vi "send_generic_trigger.vi"(7 "ensure unique insertion?":bool, 8 "error in (no error)":errorcluster, 9 "trigger type":T1, 10 "trigger variant":variant, 11 "GenericToplevelComponent in":refnum<class "GenericToplevelComponent.lvclass">) -> (0 "error out":errorcluster, 3 "GenericToplevelComponent out":refnum<class "GenericToplevelComponent.lvclass">, 4 "# elements in queue":i32, 6 "freshly inserted?":bool)   [LabVIEW 2010, in "GenericToplevelComponent.lvclass"]
uses:
  GenericToplevelComponent.lvclass
  trigger_type_enum.ctl
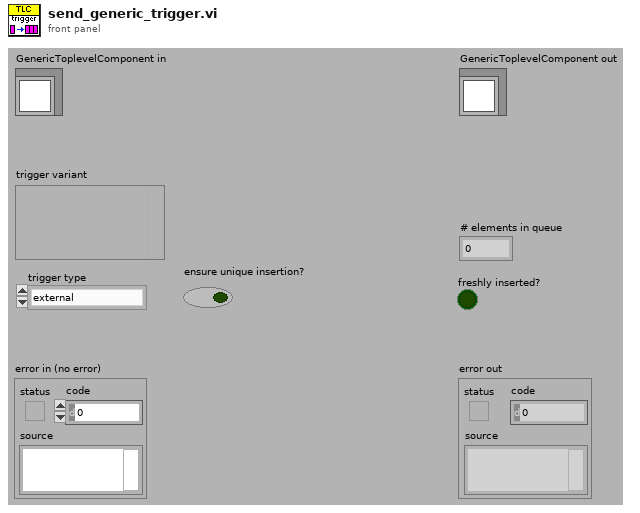
[diagram p1: front panel]
types:
  T1 = typedef "trigger_type_enum.ctl" = enum8{"external", "internal", "common"}
  T2 = typedef "top-level_component_type_enum.ctl" = enum16{"undefined", "ImagingMode", "ScanHead", "DAQ", "ImageAssembler", "Display", "DataCollection", "Analyser", "Stimulator", "ExperimentController", "Instrument", "Stage"}
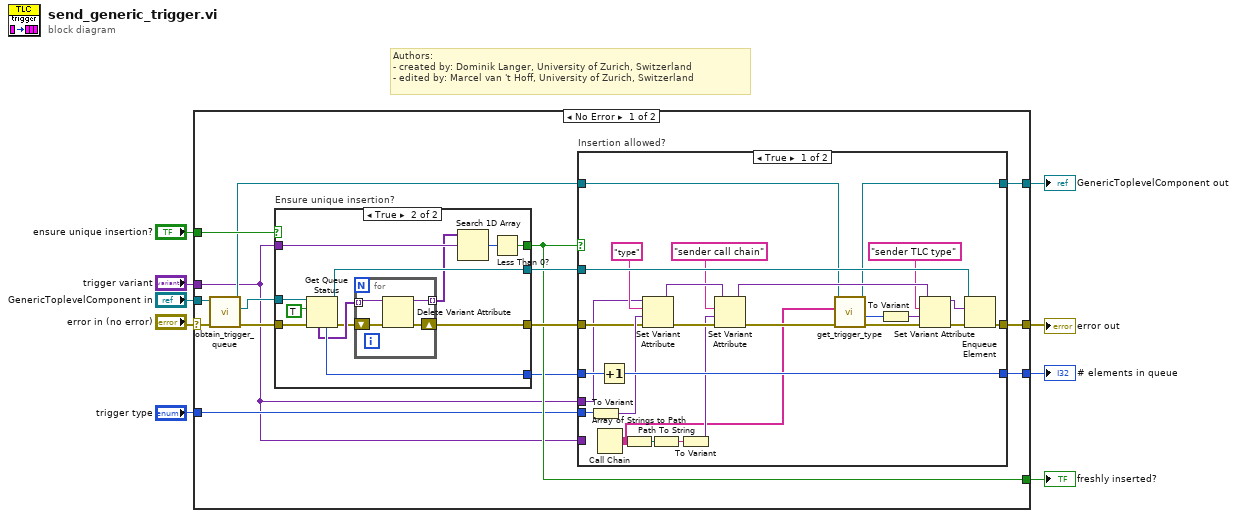
[diagram p0: block diagram]
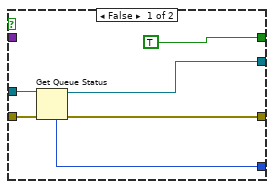
[diagram p2: hidden frame]
diagram:
  # "Authors: \n- created by: Dominik Langer, University of Zurich, Switzerland\n- edited by: Marcel van 't Hoff, University of Zurich, Switzerland"
  n1 = case shown="No Error" "error in (no error)" {
    selector: "error in (no error)" -> [w21 w77]
    tunnel: [w22 w77] -> w4
    tunnel: [w11 w76] -> w3
    tunnel: "GenericToplevelComponent in" -> [w18 w76]
    tunnel: "ensure unique insertion?" -> [w17 _]
    tunnel: "trigger type" -> [w13 _]
    tunnel: "trigger variant" -> [w10 _]
    tunnel: [w15 _] -> w2
    tunnel: [w19 _] -> w1
    frame No Error {
      n2 = call-dynamic "obtain_trigger_queue.vi"("error in (no error)"=w21, "GenericPlugin in"=w18) -> ("error out"=w14:errorcluster, "trigger queue"=w20:refnum<queue>, "GenericPlugin out"=w12:refnum<class "GenericToplevelComponent.lvclass">)  [unwired: 7 in]
      n3 = case "Ensure unique insertion?" shown="True" w17 {
        tunnel: [w27 w31] -> w24
        tunnel: [w26 w42] -> w23
        tunnel: w14 -> [w30 w40]
        tunnel: w20 -> [w29 w39]
        tunnel: [w28 w38] -> w16
        tunnel: [TRUE w35] -> w19
        tunnel: w10 -> [_ w37]
        frame False {
          n4 = Get Queue Status(queue=w29, error in (no error)=w30) -> (queue out=w26:refnum<queue>, error out=w27:errorcluster, # elements in queue=w28:i32)  [unwired: 1 in, 5 out]
        }
        frame True {
          n5 = Get Queue Status(queue=w39, return elements? (F)=TRUE, error in (no error)=w40) -> (queue out=w42:refnum<queue>, error out=w33:errorcluster, # elements in queue=w38:i32, elements=w34:variant[])  [unwired: 4 out]
          n6 = for {
            tunnel: w34 -> [w44] mode=indexing
            shift-right: [w45] -> w31
            shift-left: w33 -> [w46]
            tunnel: [w43] -> w32 mode=indexing
            n7 = Delete Variant Attribute(4:w46, 7:w44) -> (0:w45:errorcluster, 3:w43:variant)  [unwired: 1 in, 1 out]
          }
          n8 = Search 1D Array(1D array=w32, element=w37) -> (index of element=w36:i32)  [unwired: 1 out]
          n9 = Less Than 0?(x=w36) -> (x < 0?=w35:bool)
        }
      }
      n10 = case "Insertion allowed?" shown="True" w19 {
        tunnel: [w72 w75] -> w22
        tunnel: w24 -> [w61 w75]
        tunnel: w23 -> [w71 _]
        tunnel: w10 -> [w60 _]
        tunnel: w16 -> [w70 w74]
        tunnel: [w69 w74] -> w15
        tunnel: w13 -> [w57 _]
        tunnel: w12 -> [w48 w73]
        tunnel: [w52 w73] -> w11
        tunnel: w10 -> [_ _]
        frame True {
          n11 = To Variant(anything=w57) -> (Variant=w68:variant)
          n12 = Call Chain() -> (call chain=w47:string[])
          n13 = Increment(x=w70) -> (x+1=w69:i32)
          n14 = Array of Strings to Path(0:w47) -> (2:w65:path)  [unwired: 1 in]
          n15 = Set Variant Attribute(Variant=w60, name="type", value=w68, error in=w61) -> (Variant out=w66:variant, error out=w54:errorcluster)  [unwired: 1 out]
          n16 = Path To String(path=w65) -> (string=w64:string)
          n17 = To Variant(anything=w64) -> (Variant=w53:variant)
          n18 = Set Variant Attribute(Variant=w66, name="sender call chain", value=w53, error in=w54) -> (Variant out=w63:variant, error out=w49:errorcluster)  [unwired: 1 out]
          n19 = call-dynamic "get_trigger_type.vi"("error in (no error)"=w49, "call chain"=w47, "GenericToplevelComponent in"=w48) -> ("error out"=w51:errorcluster, "TLC type out"=w50:T2, "GenericToplevelComponent out"=w52:refnum<class "GenericToplevelComponent.lvclass">)  [unwired: 3 in, 3 out]
          n20 = To Variant(anything=w50) -> (Variant=w55:variant)
          n21 = Set Variant Attribute(Variant=w63, name="sender TLC type", value=w55, error in=w51) -> (Variant out=w59:variant, error out=w62:errorcluster)  [unwired: 1 out]
          n22 = Enqueue Element(queue=w71, element=w59, error in (no error)=w62) -> (error out=w72:errorcluster)  [unwired: 3 out]
        }
        frame False {
        }
      }
    }
    frame Error {
    }
  }
  "error out" <- w4
  "GenericToplevelComponent out" <- w3
  "# elements in queue" <- w2
  "freshly inserted?" <- w1
